vi "Self-Test.vi"(8 "error in (no error)":errorcluster, 10 "Device Number":u8=1, 11 "VISA resource name":refnum<visa-resource-name>) -> (0 "error out":errorcluster, 1 "Self-Test Result Message":string, 2 "Self-Test Result Code":i32, 3 "VISA resource name out":refnum<visa-resource-name>)   [LabVIEW 2020, in "ZaberTSeries.lvlib"]
doc: "Runs the instrument's self-test routine and returns the test results."
uses:
  ZaberTSeries.lvlib
  Request.ctl
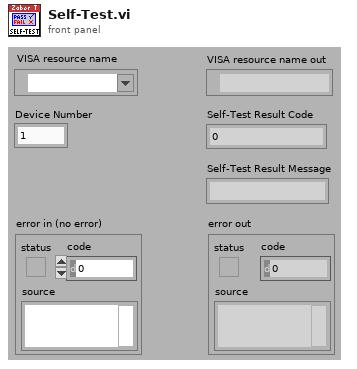
[diagram p1: front panel]
types:
  T1 = typedef "ZaberTSeries.lvlib/Request.ctl" = cluster{"Device Number":u8, "Command":u8, "Data":i32, "Response Count":i32}
  T2 = typedef "ZaberTSeries.lvlib/Response.ctl" = cluster{"Device Number":u8, "Command":u8, "Data":i32}
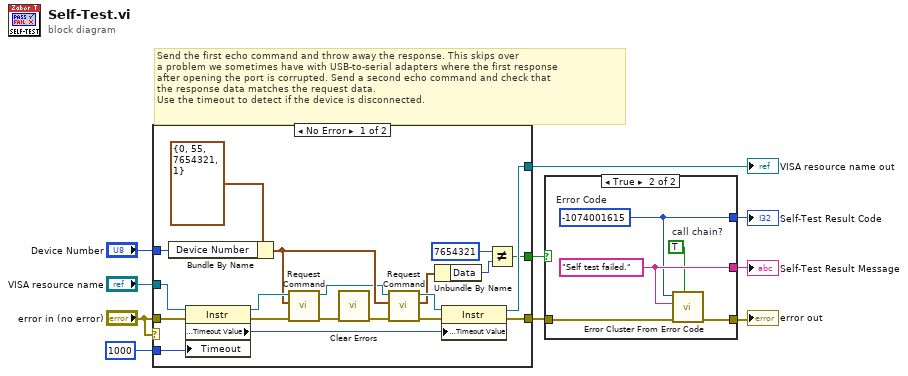
[diagram p0: block diagram]
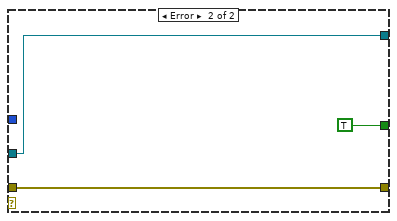
[diagram p2: hidden frame]
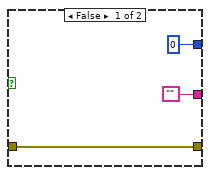
[diagram p3: hidden frame]
diagram:
  # "Send the first echo command and throw away the response. This skips over\na problem we sometimes have with USB-to-serial adapters where the first response\nafter opening the port is corrupted. Send a second echo command and check that\nthe response data matches the request data.\nUse the timeout to detect if the device is disconnected."
  n1 = case shown="No Error" "error in (no error)" {
    tunnel: "Device Number" -> [w29 _]
    tunnel: "error in (no error)" -> [w26 w32]
    tunnel: "VISA resource name" -> [w25 w33]
    tunnel: [w22 w33] -> w7
    tunnel: [w21 w32] -> w4
    tunnel: [w20 TRUE] -> w3
    tunnel: u32 1000 ("General Settings:Timeout Value") -> [w19 _]
    frame No Error {
      n2 = Bundle By Name(cluster=T1 {"Device Number"=0, "Command"=55, "Data"=7654321, "Response Count"=1} ("Request"), "Device Number"=w29) -> (w15:T1)
      n3 = property class="Instr"(reference=w25, error in=w26, "Timeout"=w19) -> (reference out=w24:refnum<visa-resource-name>, error out=w23:errorcluster, "General Settings:Timeout Value"=w18:u32)
      n4 = call "Request Command.vi"("error in (no error)"=w23, "Request"=w15, "VISA resource name"=w24) -> ("error out"=w17:errorcluster, "VISA resource name out"=w14:refnum<visa-resource-name>)  [unwired: 5 in, 2 out]
      n5 = call "Clear Errors.vi"("error in (no error)"=w17) -> ("error out"=w16:errorcluster)  [unwired: 5 in, 1 out]
      n6 = call "Request Command.vi"("error in (no error)"=w16, "Request"=w15, "VISA resource name"=w14) -> ("error out"=w12:errorcluster, "First Response"=w11:T2, "VISA resource name out"=w13:refnum<visa-resource-name>)  [unwired: 5 in, 1 out]
      n7 = Unbundle By Name(w11) -> ("Data"=w28:i32)
      n8 = property class="Instr"(reference=w13, error in=w12, "General Settings:Timeout Value"=w18) -> (reference out=w22:refnum<visa-resource-name>, error out=w21:errorcluster)
      n9 = Not Equal?(x=7654321, y=w28) -> (x != y?=w20:bool)
    }
    frame Error {
    }
  }
  "VISA resource name out" <- w7
  n10 = case shown="True" w3 {
    tunnel: [0 ("Self-Test Result Code") w40] -> w8
    tunnel: ["" ("Self-Test Result Message") w41] -> w6
    tunnel: [w34 w38] -> w5
    tunnel: w4 -> [w34 w37]
    frame False {
    }
    frame True {
      w39 = TRUE  # call chain?
      w41 = "Self test failed." ("Self-Test Result Message")
      w40 = -1074001615  # Error Code
      n11 = call "Error Cluster From Error Code.vi"("show call chain? (False)"=w39, "error in (no error)"=w37, "error message (\"\")"=w41, "error code (0)"=w40) -> ("error out"=w38:errorcluster)  [unwired: 5 in]
    }
  }
  "error out" <- w5
  "Self-Test Result Message" <- w6
  "Self-Test Result Code" <- w8
